vi "MAST_Gage_Acquisition_mod.vi"() -> ()   [LabVIEW 2017]
uses:
  <instrlib>/niHWS/nihws.llb/niHWS Open File Permissions ID.ctl
  <instrlib>/niHWS/nihws.llb/niHWS Set Wfm DBL Attribute ID.ctl
  <instrlib>/niHWS/nihws.llb/niHWS Set Wfm DBL Attribute.vi
  <instrlib>/niHWS/nihws.llb/niHWS Write Analog I16.vi
panel:
  out "Status 2":i32
  out "Error String":string
  in  "One run":bool=TRUE
  out "Waveform Graph":cluster{dbl, dbl, "Data in Volts":i16[]}(graph) caption="Page 1  of  1"
  in  "Save HWS to:":path=path "C:/Users/plasma/Desktop/test.hws"
  in  "Length":dbl=261120.0 min=128.0 max=261120.0
  in  "Start Point":dbl min=-10000000000.0 max=26112000000.0 step=16.0
  in  "Trigger":T1={"Slope"=0, "Level"=20, "Source"=0, "External Range"=2000, "External Coupling"=0, "External"=FALSE, "Disable"=FALSE, "External Impedance"=1} {"External Impedance" items=["50 Ohm", "HiZ"]; "External Coupling" items=["DC", "AC"]; "External Range" min=2000 max=10000 step=8000; "Slope" items=["Rising", "Falling"]; "Level" min=-100 max=100; "Source" min=0 max=64 step=1}
  in  "stop":bool
  in  "Page Size":dbl=32640.0 min=4080.0 step=4080.0
  out "Status":string
  in  "Channels":T2(array[cluster])=[{"Coupling"=0, "Differential Input"=FALSE, "Direct-to-ADC"=FALSE, "Range"=2000, "Impedance"=50, "DC Offset"=0, "Filter"=0}] {"Impedance" min=50 max=1000000 step=999950; "Coupling" items=["DC", "AC"]}
  in  "Acquisition":T3={"Sample Rate"=10000000.0, "Mode"=0, "Depth"=261120.0, "Acquisiton time(s)"=1.0000016, "Trigger Timeout(s)"=10.0, "Trigger Holdoff"=0.0, "Trigger Delay"=0.0, "Clock mode"=enum."Internal"} {"Acquisiton time(s)" min=1.6e-05 max=200.0 step=0.001 format="%_5p"; "Trigger Delay" min=0.0 step=1e-06; "Trigger Holdoff" min=0.0 step=128.0; "Depth" min=16.0 step=16.0; "Mode" items=["Single", "Dual", "Quad", "Octal"]; "Sample Rate" format="%.0p"}
  out "System Name":string
  out "Channel Count":u16
  out "Board Count":u16
  out "System Count":i32
  # "Fetching splitting parameters"
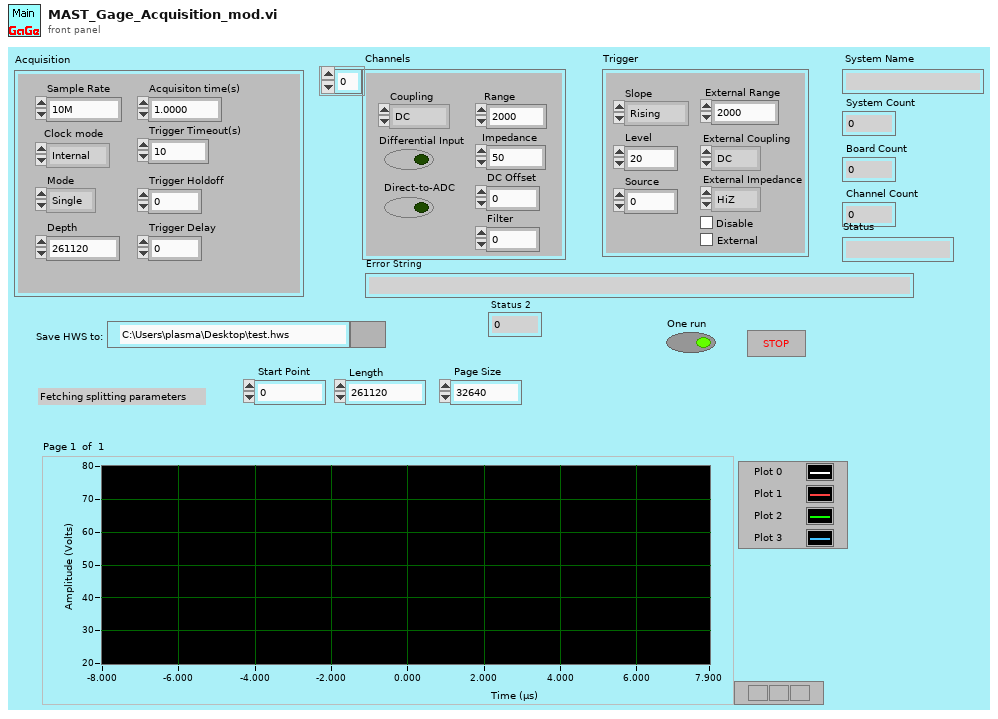
[diagram p1: front panel]
types:
  T1 = cluster{"Slope":u16, "Level":i32, "Source":i32, "External Range":u32, "External Coupling":u16, "External":bool, "Disable":bool, "External Impedance":u16}
  T2 = cluster{"Coupling":u16, "Differential Input":bool, "Direct-to-ADC":bool, "Range":u32, "Impedance":u32, "DC Offset":i32, "Filter":i32}[]
  T3 = cluster{"Sample Rate":dbl, "Mode":u16, "Depth":dbl, "Acquisiton time(s)":dbl, "Trigger Timeout(s)":dbl, "Trigger Holdoff":dbl, "Trigger Delay":dbl, "Clock mode":enum16{"Internal", "External", "Reference"}}
  T4 = typedef "niHWS Open File Permissions ID.ctl" = enum32{"Read Only", "Read/Write Existing", "Read/Write/Create New", "Read/Write/Create New Always"}
  T5 = cluster{"Handle":u32, "Sample size":u32, "Resolution":i32, "Offset":i32, "Channels":u32, "Boards":u32}
  T6 = cluster{"Coupling":u16, "Differential Input":bool, "Direct-to-ADC":bool, "Range":u32, "Impedance":u32, "DC Offset":i32, "Filter":i32}
  T7 = cluster{string, "Differential Input":bool, "Direct-to-ADC":bool, "Range":u32, "Impedance":u32, "DC Offset":i32, "Filter":i32}
  T8 = cluster{"RingText.Text":string, "Level":i32, "Source":i32, "External Range":u32, "RingText.Text":string, "External":bool, "Disable":bool, "RingText.Text":string}
  T9 = cluster{"RingText.Text":string, "Level":i32, "Source":i32, "External Range":u32, "RingText.Text":string, "External":bool, "Disable":bool, "RingText.Text":string}[]
  T10 = cluster{"Sample Rate":dbl, "Clock mode":enum16{"Internal", "External", "Reference"}, "RingText.Text":string, dbl, dbl, dbl, "Trigger Holdoff":dbl, dbl}
  T11 = cluster{"Handle":u32, "Sample Size":u32, "Resolution":i32, "Offset":i32, "Channels":u32, "Boards":u32}
  T12 = typedef "niHWS Set Wfm DBL Attribute ID.ctl" = u32
  T13 = cluster{dbl, dbl, "Data before\n conversion":i16[]}
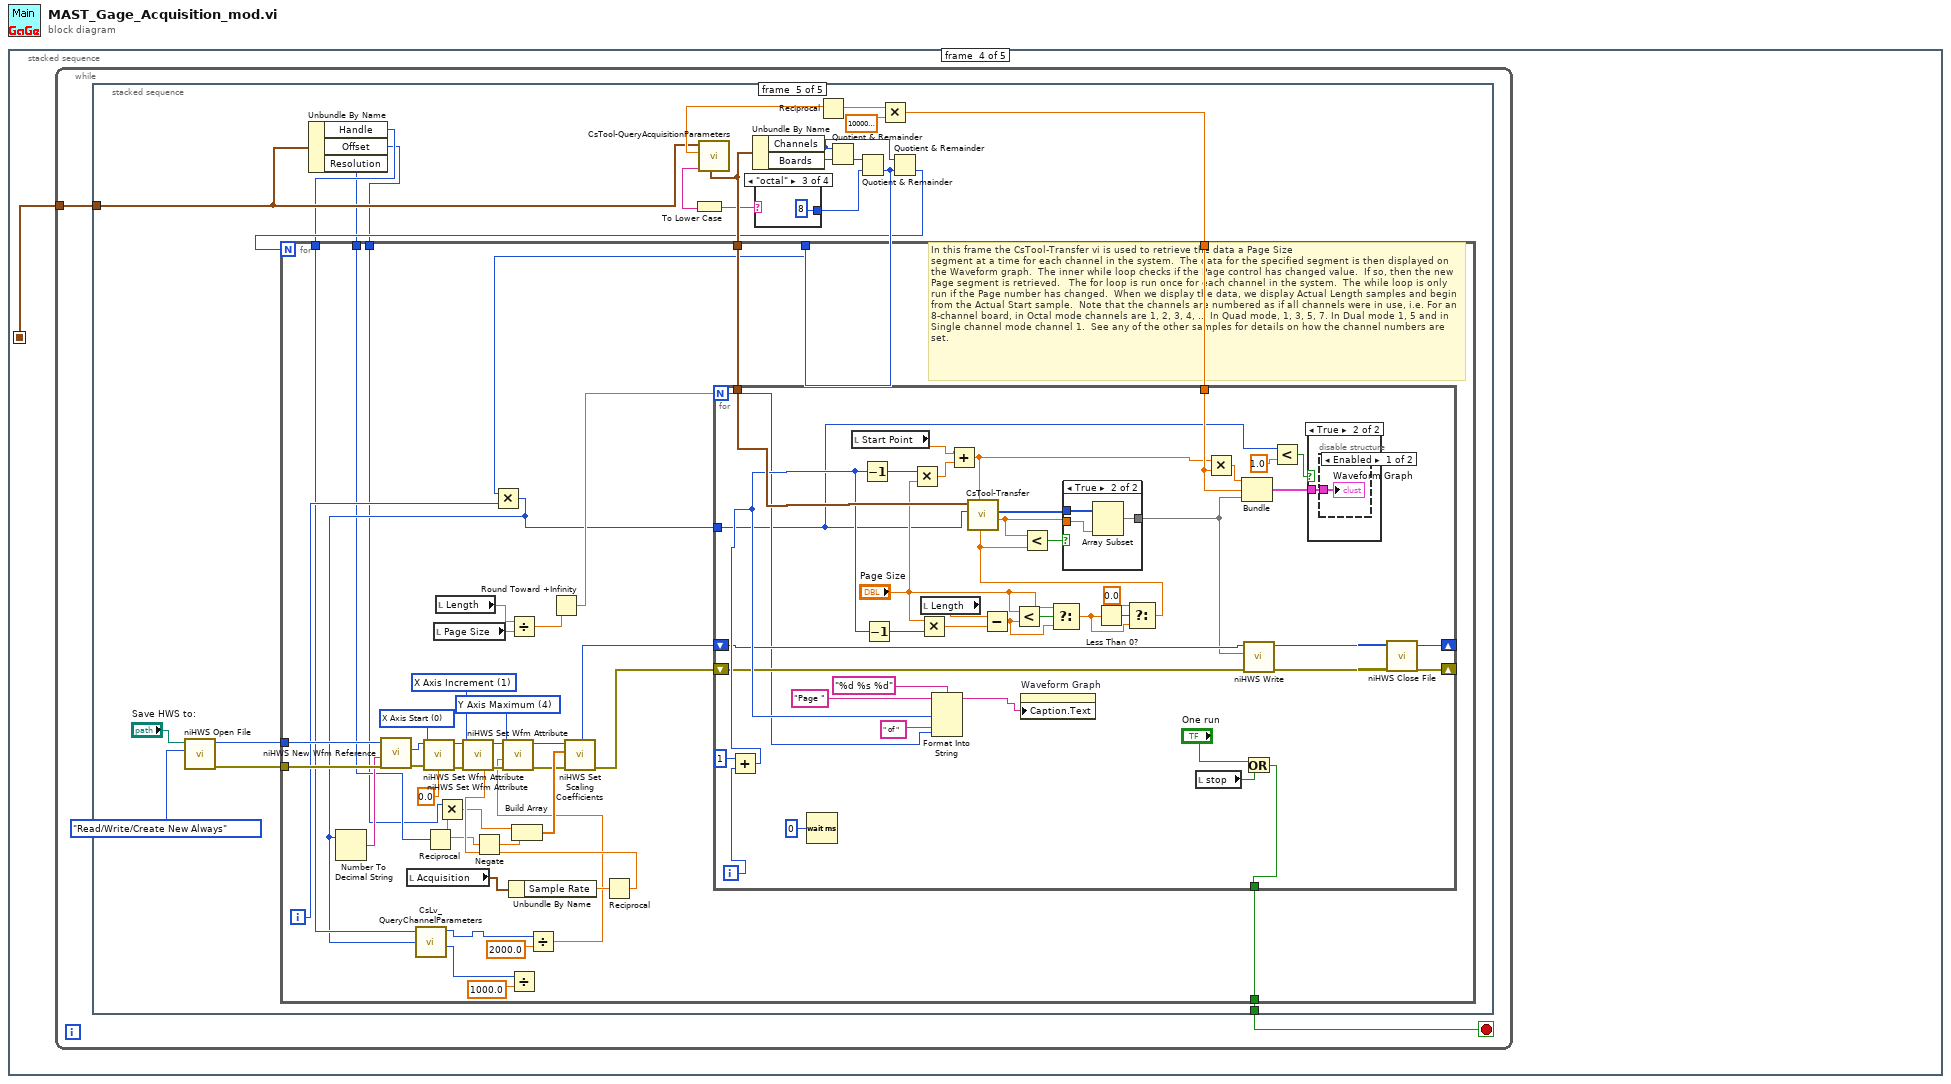
[diagram p0: block diagram]
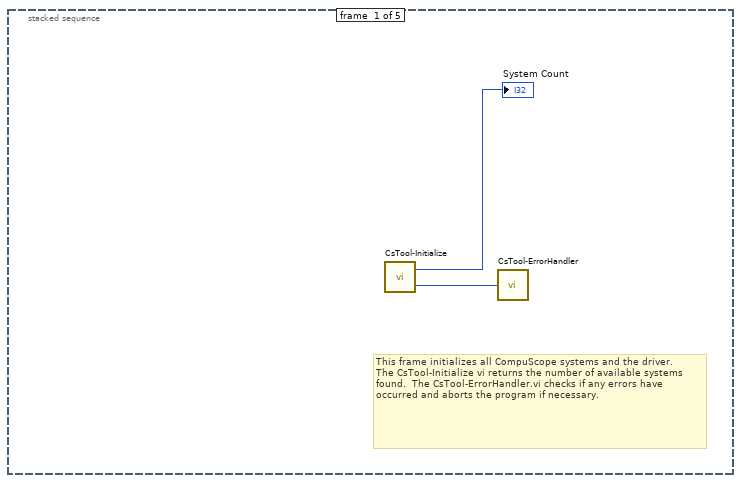
[diagram p2: hidden frame]
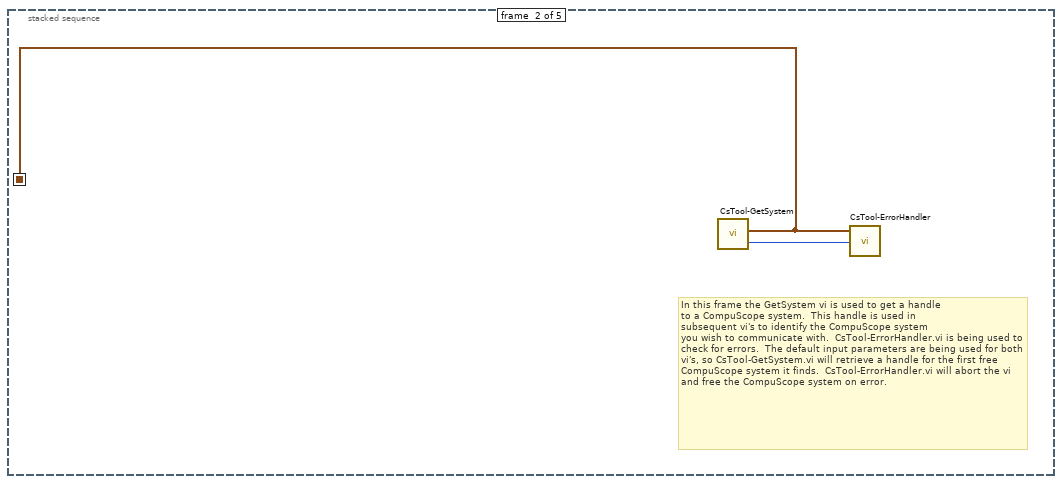
[diagram p3: hidden frame]
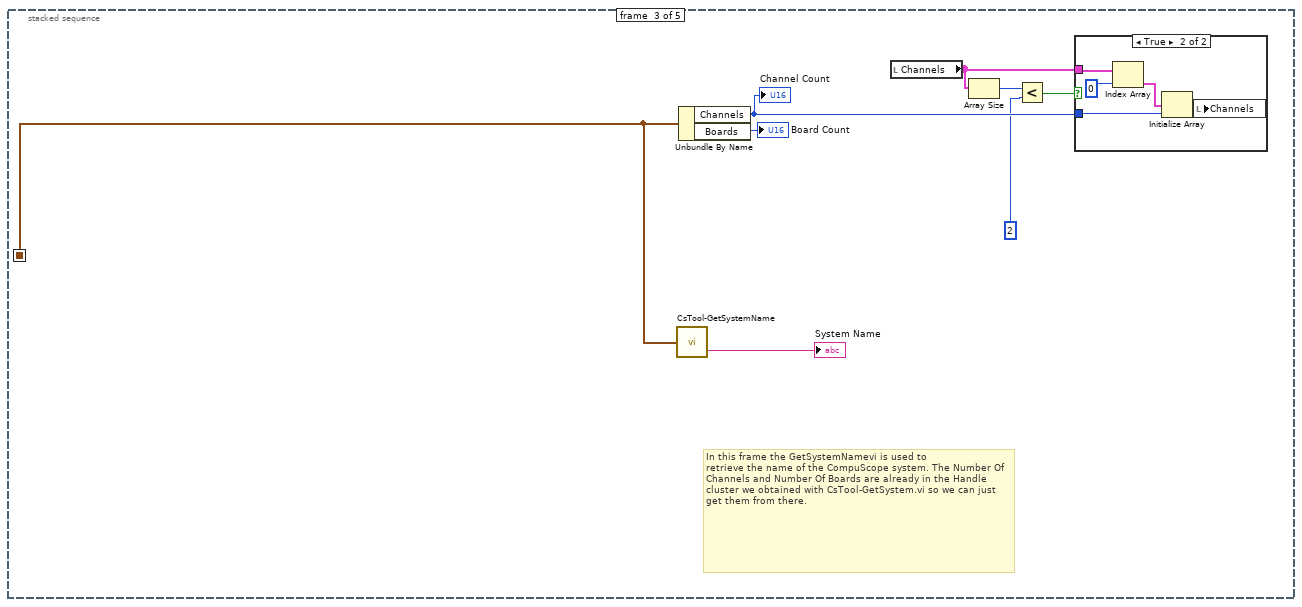
[diagram p4: hidden frame]
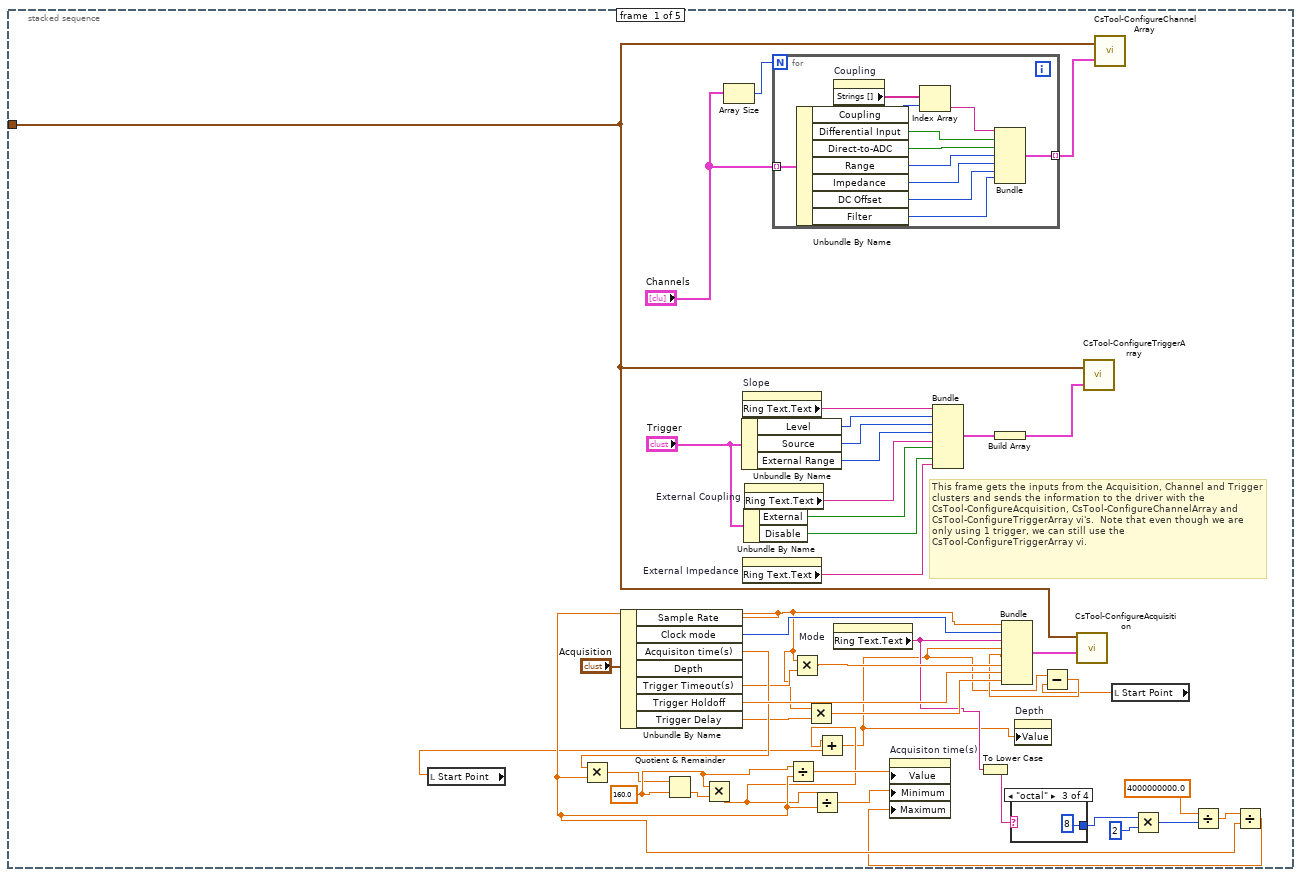
[diagram p6: hidden frame]
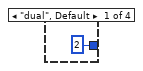
[diagram p7: hidden frame]
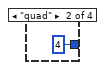
[diagram p8: hidden frame]
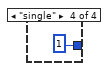
[diagram p9: hidden frame]
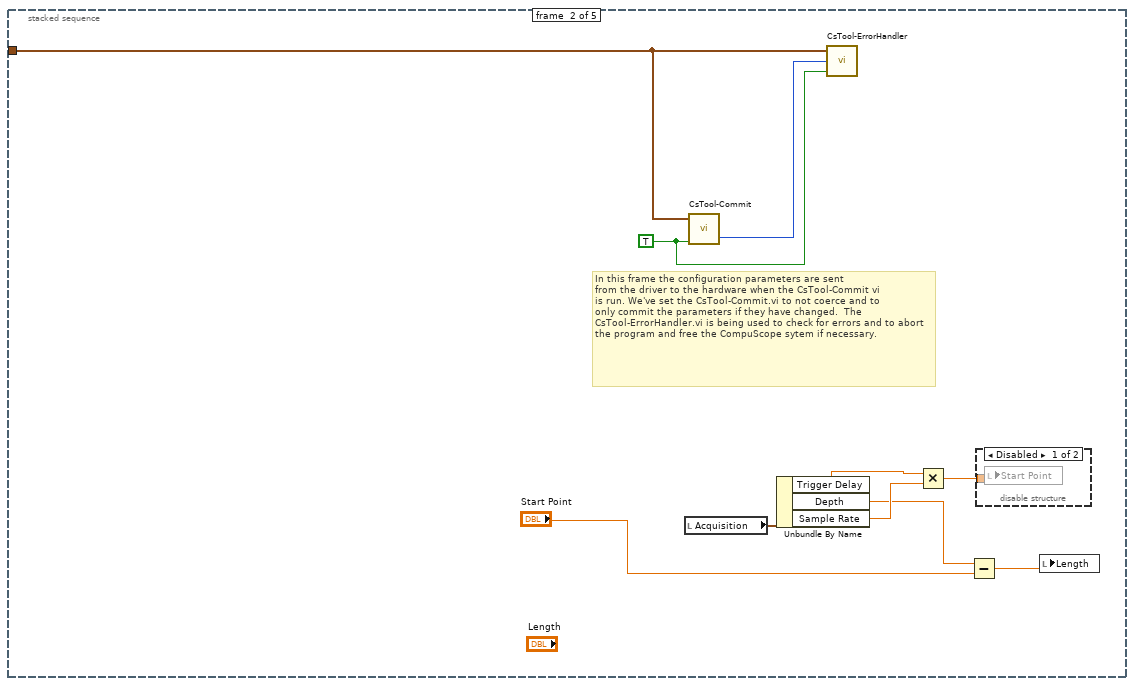
[diagram p10: hidden frame]
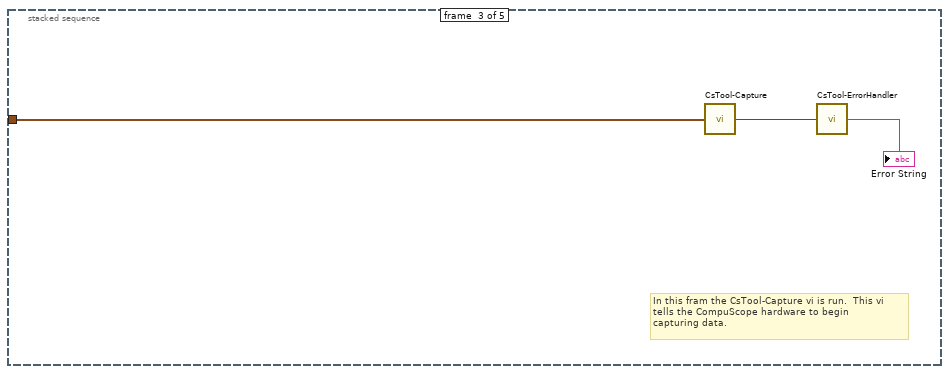
[diagram p12: hidden frame]
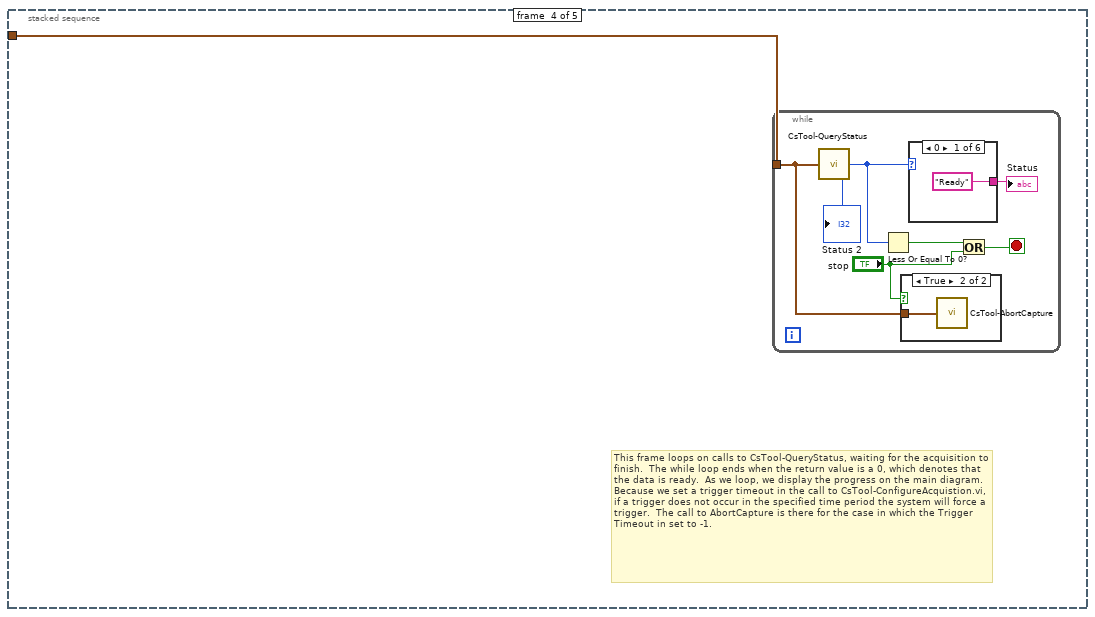
[diagram p13: hidden frame]
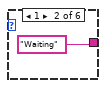
[diagram p15: hidden frame]
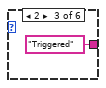
[diagram p16: hidden frame]
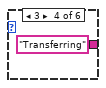
[diagram p17: hidden frame]
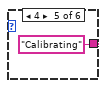
[diagram p18: hidden frame]
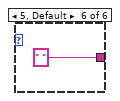
[diagram p19: hidden frame]
diagram:
  n1 = stacked-sequence {
    seq-local: [_ w3 _ _ _] -> [_ _ w11 w18 w225]
    frame #0 {
      # "This frame initializes all CompuScope systems and the driver.\nThe CsTool-Initialize vi returns the number of available systems found.  The CsTool-ErrorHandler.vi checks if any errors have occurred and aborts the program if necessary."
      n2 = call <userlib>:"CsTool-Initialize.vi"() -> ("Error Code"=w2:i32, "Number Of Systems"=→"System Count":i32)
      n3 = call <userlib>:"CsTool-ErrorHandler.vi"("Error Code"=w2) -> ()  [unwired: 2 in, 1 out]
    }
    frame #1 {
      # "In this frame the GetSystem vi is used to get a handle \nto a CompuScope system.  This handle is used in \nsubsequent vi's to identify the CompuScope system \nyou wish to communicate with.  CsTool-ErrorHandler.vi is being used to check for errors.  The default input parameters are being used for both vi's, so CsTool-GetSystem.vi will retrieve a handle for the first free CompuScope system it finds.  CsTool-ErrorHandler.vi will abort the vi and free the CompuScope system on error."
      n4 = call <userlib>:"CsTool-GetSystem.vi"() -> ("Error Code"=w4:i32, "Handle Cluster"=w3:T5)  [unwired: 4 in]
      n5 = call <userlib>:"CsTool-ErrorHandler.vi"("Error Code"=w4, "Handle Cluster"=w3) -> ()  [unwired: 1 in, 1 out]
    }
    frame #2 {
      # "In this frame the GetSystemNamevi is used to\nretrieve the name of the CompuScope system. The Number Of Channels and Number Of Boards are already in the Handle cluster we obtained with CsTool-GetSystem.vi so we can just get them from there."
      n6 = call <userlib>:"CsTool-GetSystemName.vi"("Handle Cluster"=w11) -> ("System Name"=→"System Name":string)  [unwired: 1 out]
      n7 = Unbundle By Name(w11) -> ("Channels"=w10:u32, "Boards"=→"Board Count":u32)
      "Channel Count" <- w10
      n8 = local read "Channels"() -> (w7:T2)
      n9 = Array Size(array=w7) -> (size(s)=w8:i32)
      n10 = Less?(x=w8, y=2) -> (x < y?=w9:bool)
      n11 = case shown="True" w9 {
        tunnel: w7 -> [_ w15]
        tunnel: w10 -> [_ w13]
        frame False {
        }
        frame True {
          n12 = Index Array(array=w15, index=0) -> (element=w14:T6)
          n13 = Initialize Array(w14, w13) -> (w16:T2)
          n14 = local write "Channels"(w16) -> ()
        }
      }
    }
    frame #3 {
      n15 = while {
        tunnel: w18 -> [w20]
        stop <- w19 stop-if-true
        n16 = stacked-sequence {
          tunnel: w20 -> [w59 w86 w91 w93 w110]
          tunnel: [_ _ _ _ w123] -> w19
          frame #0 {
            w43 = 160.0 ("y")
            # "This frame gets the inputs from the Acquisition, Channel and Trigger clusters and sends the information to the driver with the CsTool-ConfigureAcquisition, CsTool-ConfigureChannelArray and CsTool-ConfigureTriggerArray vi's.  Note that even though we are only using 1 trigger, we can still use the CsTool-ConfigureTriggerArray vi."
            n17 = local read "Start Point"() -> (w24:dbl)
            n18 = Unbundle By Name("Acquisition") -> ("Sample Rate"=w29:dbl, "Clock mode"=w45:enum16{"Internal", "External", "Reference"}, "Acquisiton time(s)"=w42:dbl, "Trigger Timeout(s)"=w38:dbl, "Trigger Holdoff"=w48:dbl, "Trigger Delay"=w36:dbl)  [unwired: 1 out]
            n19 = Multiply(x=w42, y=w29) -> (x*y=w41:dbl)
            n20 = Quotient & Remainder(x=w41, y=w43) -> (floor(x/y)=w44:dbl)  [unwired: 1 out]
            n21 = Multiply(x=w43, y=w44) -> (x*y=w25:dbl)
            n22 = Array Size(array="Channels") -> (size(s)=w62:i32)
            n23 = Unbundle By Name("Trigger") -> ("Level"=w57:i32, "Source"=w55:i32, "External Range"=w54:u32)
            n24 = property on="Slope" class="Ring (strict)"() -> ("Ring Text.Text"=w51:string)  [unwired: 2 in, 2 out]
            n25 = property on="External Impedance" class="Ring (strict)"() -> ("Ring Text.Text"=w49:string)  [unwired: 2 in, 2 out]
            n26 = Unbundle By Name("Trigger") -> ("External"=w56:bool, "Disable"=w53:bool)
            n27 = property on="External Coupling" class="Ring (strict)"() -> ("Ring Text.Text"=w50:string)  [unwired: 2 in, 2 out]
            n28 = for {
              N: w62 -> [_]
              tunnel: "Channels" -> [w74] mode=indexing
              tunnel: [w75] -> w60 mode=indexing
              n29 = Unbundle By Name(w74) -> ("Coupling"=w78:u16, "Differential Input"=w73:bool, "Direct-to-ADC"=w72:bool, "Range"=w71:u32, "Impedance"=w70:u32, "DC Offset"=w69:i32, "Filter"=w68:i32)
              n30 = property on="Coupling" class="Ring (strict)"() -> ("Strings []"=w77:string[])  [unwired: 2 in, 2 out]
              n31 = Index Array(array=w77, index=w78) -> (element=w76:string)
              n32 = Bundle(w76, "Differential Input"=w73, "Direct-to-ADC"=w72, "Range"=w71, "Impedance"=w70, "DC Offset"=w69, "Filter"=w68) -> (w75:T7)  [unwired: 1 in]
            }
            n33 = Divide(x=w43, y=w29) -> (x/y=w40:dbl)
            n34 = Multiply(x=w29, y=w38) -> (x*y=w37:dbl)
            n35 = Multiply(x=w29, y=w36) -> (x*y=w35:dbl)
            n36 = Divide(x=w25, y=w29) -> (x/y=w39:dbl)
            n37 = Add(x=w25, y=w24) -> (x+y=w22:dbl)
            n38 = property on="Mode" class="Ring (strict)"() -> ("Ring Text.Text"=w27:string)  [unwired: 2 in, 2 out]
            n39 = Bundle("RingText.Text"=w51, "Level"=w57, "Source"=w55, "External Range"=w54, "RingText.Text"=w50, "External"=w56, "Disable"=w53, "RingText.Text"=w49) -> (w47:T8)  [unwired: 1 in]
            n40 = To Lower Case(string=w27) -> (all lower case string=w26:string)
            n41 = Build Array(w47) -> (w46:T9)
            n42 = case shown="\"octal\"" w26 {
              tunnel: [2 4 8 1] -> w34
              frame "dual", Default {
              }
              frame "quad" {
              }
              frame "octal" {
              }
              frame "single" {
              }
            }
            n43 = property on="Depth" class="DigNum (strict)"("Value"=w22) -> ()  [unwired: 2 in, 2 out]
            n44 = call <userlib>:"CsTool-ConfigureTriggerArray.vi"("Triggers"=w46, "Handle Cluster"=w59) -> ()  [unwired: 1 out]
            n45 = call <userlib>:"CsTool-ConfigureChannelArray.vi"("Channels"=w60, "Handle Cluster"=w59) -> ()  [unwired: 1 out]
            n46 = local read "Start Point"() -> (w21:dbl)
            n47 = Subtract(x=w22, y=w21) -> (x-y=w23:dbl)
            n48 = Bundle("Sample Rate"=w29, "Clock mode"=w45, "RingText.Text"=w27, w22, w23, w37, "Trigger Holdoff"=w48, w35) -> (w63:T10)  [unwired: 1 in]
            n49 = call <userlib>:"CsTool-ConfigureAcquisition.vi"("Handle Cluster"=w59, "Acquisition"=w63) -> ()  [unwired: 3 in, 1 out]
            n50 = Multiply(x=w34, y=2) -> (x*y=w31:i32)
            n51 = Divide(x=4000000000.0, y=w31) -> (x/y=w30:dbl)
            n52 = Divide(x=w30, y=w29) -> (x/y=w28:dbl)
            n53 = property on="Acquisiton time(s)" class="DigNum (strict)"("Value"=w39, "Minimum"=w40, "Maximum"=w28) -> ()  [unwired: 2 in, 2 out]
          }
          frame #1 {
            w87 = TRUE
            # "In this frame the configuration parameters are sent\nfrom the driver to the hardware when the CsTool-Commit vi \nis run. We've set the CsTool-Commit.vi to not coerce and to\nonly commit the parameters if they have changed.  The CsTool-ErrorHandler.vi is being used to check for errors and to abort the program and free the CompuScope sytem if necessary."
            n54 = local read "Acquisition"() -> (w85:T3)
            n55 = call <userlib>:"CsTool-Commit.vi"("OnlyOnChange (t)"=w87, "Handle Cluster"=w86) -> ("Error Code"=w88:i32)  [unwired: 1 in, 1 out]
            n56 = Unbundle By Name(w85) -> ("Trigger Delay"=w84:dbl, "Depth"=w81:dbl, "Sample Rate"=w83:dbl)
            n57 = call <userlib>:"CsTool-ErrorHandler.vi"("StopOnError (true)"=w87, "Error Code"=w88, "Handle Cluster"=w86) -> ()  [unwired: 1 out]
            n58 = Multiply(x=w84, y=w83) -> (x*y=w82:dbl)
            n59 = Subtract(x=w81, y="Start Point") -> (x-y=w80:dbl)
            n60 = disable-structure shown="Disabled" {
              disable-tunnel: w82 -> [w89 _]
              frame Disabled {
                n61 = local write "Start Point"(w89) -> ()
              }
              frame Enabled {
              }
            }
            n62 = local write "Length"(w80) -> ()
          }
          frame #2 {
            # "In this fram the CsTool-Capture vi is run.  This vi\ntells the CompuScope hardware to begin\ncapturing data."
            n63 = call <userlib>:"CsTool-Capture.vi"("Handle Cluster"=w91) -> ("Error Code"=w92:i32)
            n64 = call <userlib>:"CsTool-ErrorHandler.vi"("Error Code"=w92) -> ("Error String"=→"Error String":string)  [unwired: 2 in]
          }
          frame #3 {
            # "This frame loops on calls to CsTool-QueryStatus, waiting for the acquisition to finish.  The while loop ends when the return value is a 0, which denotes that the data is ready.  As we loop, we display the progress on the main diagram.  Because we set a trigger timeout in the call to CsTool-ConfigureAcquistion.vi, if a trigger does not occur in the specified time period the system will force a trigger.  The call to AbortCapture is there for the case in which the Trigger Timeout in set to -1."
            n65 = while {
              tunnel: w93 -> [w95]
              stop <- w96 stop-if-true
              n66 = call <userlib>:"CsTool-QueryStatus.vi"("Handle Cluster"=w95) -> ("Status"=w99:i32)
              "Status 2" <- w99
              n67 = Less Or Equal To 0?(x=w99) -> (x <= 0?=w97:bool)
              n68 = case shown="True" "stop" {
                tunnel: w95 -> [_ w100]
                frame False {
                }
                frame True {
                  n69 = call <userlib>:"CsTool-AbortCapture.vi"("Handle Cluster"=w100) -> ()  [unwired: 1 out]
                }
              }
              n70 = case shown="0" w99 {
                tunnel: ["Ready" "Waiting" "Triggered" "Transferring" "Calibrating" " "] -> w98
                frame 0 {
                }
                frame 1 {
                }
                frame 2 {
                }
                frame 3 {
                }
                frame 4 {
                }
                frame 5, Default {
                }
              }
              "Status" <- w98
              n71 = Or(x=w97, y="stop") -> (x .or. y?=w96:bool)
            }
          }
          frame #4 {
            n72 = call <instrlib>:"niHWS Open File.vi"("permissions (0:read only)"=niHWS_Open_File_Permissions_ID."Read/Write/Create New Always", "file path"="Save HWS to:") -> ("error out"=w113:errorcluster, "file handle"=w114:u32)  [unwired: 8 in]
            n73 = Unbundle By Name(w110) -> ("Handle"=w109:u32, "Offset"=w108:i32, "Resolution"=w107:i32)
            n74 = call <userlib>:"CsTool-QueryAcquisitionParameters.vi"("Handle Cluster"=w110) -> ("Output Handle Cluster"=w128:T11, "Mode"=w117:string, "Sample Rate"=w121:dbl)  [unwired: 8 out]
            n75 = To Lower Case(string=w117) -> (all lower case string=w127:string)
            n76 = Unbundle By Name(w128) -> ("Channels"=w125:u32, "Boards"=w122:u32)
            n77 = case shown="\"octal\"" w127 {
              tunnel: [2 4 8 1] -> w116
              frame "dual", Default {
              }
              frame "quad" {
              }
              frame "octal" {
              }
              frame "single" {
              }
            }
            n78 = Reciprocal(x=w121) -> (1/x=w120:dbl)
            n79 = Quotient & Remainder(x=w125, y=w122) -> (floor(x/y)=w126:u32)  [unwired: 1 out]
            n80 = Quotient & Remainder(x=w126, y=w116) -> (floor(x/y)=w124:u32)  [unwired: 1 out]
            n81 = Multiply(x=w120, y=1000000.0) -> (x*y=w118:dbl)
            n82 = Quotient & Remainder(x=w125, y=w124) -> (floor(x/y)=w111:u32)  [unwired: 1 out]
            n83 = for {
              N: w111 -> [_]
              tunnel: w128 -> [w172]
              tunnel: w124 -> [w171]
              tunnel: [w170] -> w123
              tunnel: w118 -> [w169]
              tunnel: w114 -> [w164]
              tunnel: w113 -> [w163]
              tunnel: w109 -> [w142]
              tunnel: w108 -> [w132]
              tunnel: w107 -> [w133]
              i -> [w151]
              w143 = T12 4 items=["X Axis Start"=0, "X Axis Increment"=1, "Y Axis Minimum"=3, "Y Axis Maximum"=4] ("attribute ID")
              w156 = T12 1 items=["X Axis Start"=0, "X Axis Increment"=1, "Y Axis Minimum"=3, "Y Axis Maximum"=4] ("attribute ID")
              w161 = T12 0 items=["X Axis Start"=0, "X Axis Increment"=1, "Y Axis Minimum"=3, "Y Axis Maximum"=4] ("attribute ID")
              # "In this frame the CsTool-Transfer vi is used to retrieve the data a Page Size \nsegment at a time for each channel in the system.  The data for the specified segment is then displayed on the Waveform graph.  The inner while loop checks if the Page control has changed value.  If so, then the new Page segment is retrieved.   The for loop is run once for each channel in the system.  The while loop is only run if the Page number has changed.  When we display the data, we display Actual Length samples and begin from the Actual Start sample.  Note that the channels are numbered as if all channels were in use, i.e. For an 8-channel board, in Octal mode channels are 1, 2, 3, 4, ... In Quad mode, 1, 3, 5, 7. In Dual mode 1, 5 and in Single channel mode channel 1.  See any of the other samples for details on how the channel numbers are set."
              n84 = local read "Acquisition"() -> (w150:T3)
              n85 = Reciprocal(x=w133) -> (1/x=w130:dbl)
              n86 = local read "Page Size"() -> (w166:dbl)
              n87 = local read "Length"() -> (w168:dbl)
              n88 = Multiply(x=w132, y=w130) -> (x*y=w131:dbl)
              n89 = Negate(x=w130) -> (-x=w129:dbl)
              n90 = Multiply(x=w171, y=w151) -> (x*y=w141:u32)
              n91 = Number To Decimal String(number=w141) -> (decimal integer string=w152:string)  [unwired: 1 in]
              n92 = call <instrlib>:"niHWS New Wfm Reference.vi"("error in (no error)"=w163, "waveform name (empty)"=w152, "file handle in"=w164) -> ("error out"=w159:errorcluster, "waveform reference"=w162:u32)  [unwired: 6 in, 1 out]
              n93 = call <userlib>:"CsLv_QueryChannelParameters.vi"("Channel"=w141, "Handle"=w142) -> ("DC Offset (mV)"=w136:i32, "Input Range (mV)"=w139:u32)  [unwired: 5 out]
              n94 = call-poly <instrlib>:"niHWS Set Wfm Attribute.vi"("error in (no error)"=w159, "attribute value"=0.0, "attribute ID"=w161, "waveform reference in"=w162) -> ("error out"=w158:errorcluster, "waveform reference out"=w157:u32)  [unwired: 6 in]
              n95 = Divide(x=w168, y=w166) -> (x/y=w167:dbl)
              n96 = Unbundle By Name(w150) -> ("Sample Rate"=w149:dbl)
              n97 = Divide(x=w136, y=1000.0) -> ()  [unwired: 1 out]
              n98 = Build Array(w131, w129) -> (w155:dbl[])
              n99 = Divide(x=w139, y=2000.0) -> (x/y=w138:dbl)
              n100 = Round Toward +Infinity(x=w167) -> (ceil(x): smallest int >= x=w165:dbl)
              n101 = Reciprocal(x=w149) -> (1/x=w148:dbl)
              n102 = call-poly <instrlib>:"niHWS Set Wfm Attribute.vi"("error in (no error)"=w158, "attribute value"=w148, "attribute ID"=w156, "waveform reference in"=w157) -> ("error out"=w147:errorcluster, "waveform reference out"=w145:u32)  [unwired: 6 in]
              n103 = call-poly <instrlib>:"niHWS Set Wfm Attribute.vi"("error in (no error)"=w147, "attribute value"=w138, "attribute ID"=w143, "waveform reference in"=w145) -> ("error out"=w146:errorcluster, "waveform reference out"=w144:u32)  [unwired: 6 in]
              n104 = call <instrlib>:"niHWS Set Scaling Coefficients.vi"("error in (no error)"=w146, "coefficient array"=w155, "waveform reference in"=w144) -> ("error out"=w153:errorcluster, "waveform reference out"=w154:u32)  [unwired: 7 in]
              n105 = for {
                N: w165 -> [w176]
                tunnel: w172 -> [w207]
                tunnel: w169 -> [w209]
                tunnel: [w186] -> w170
                shift-right: [w180] -> w135
                shift-left: w154 -> [w182]
                shift-right: [w179] -> w134
                shift-left: w153 -> [w181]
                tunnel: w141 -> [w173]
                i -> [w185]
                n106 = Add(x=1, y=w185) -> (x+y=w184:i32)
                n107 = Wait (ms)(milliseconds to wait=u32 0) -> ()  [unwired: 1 out]
                n108 = local read "Start Point"() -> (w187:dbl)
                n109 = Decrement(x=w184) -> (x-1=w200:i32)
                n110 = Decrement(x=w184) -> (x-1=w191:i32)
                n111 = Multiply(x=w200, y="Page Size") -> (x*y=w199:dbl)
                n112 = Multiply(x="Page Size", y=w191) -> (x*y=w197:dbl)
                n113 = local read "Length"() -> (w198:dbl)
                n114 = Format Into String(format string="%d %s %d", initial string="Page ", w184, " of ", w176) -> (resulting string=w177:string)  [unwired: 1 in, 1 out]
                n115 = Add(x=w187, y=w199) -> (x+y=w203:dbl)
                n116 = Subtract(x=w198, y=w197) -> (x-y=w195:dbl)
                n117 = Less?(x="Page Size", y=w195) -> (x < y?=w196:bool)
                n118 = property on="Waveform Graph" class="WFGraph (strict)"("Caption.Text"=w177) -> ()  [unwired: 2 in, 2 out]
                n119 = Select(t="Page Size", s=w196, f=w195) -> (s? t:f=w192:dbl)
                n120 = Less Than 0?(x=w192) -> (x < 0?=w194:bool)
                n121 = Select(t=0.0, s=w194, f=w192) -> (s? t:f=w189:dbl)
                n122 = call <userlib>:"CsTool-Transfer.vi"("Length (4096)"=w189, "Start (0)"=w203, "Channel (0)"=w173, "Handle Cluster"=w207) -> ("Actual Length"=w188:dbl, "Data before\n conversion"=w201:i16[])  [unwired: 2 in, 2 out]
                n123 = Less?(x=w188, y=w189) -> (x < y?=w202:bool)
                n124 = case shown="True" w202 {
                  tunnel: w201 -> [w216 w219]
                  tunnel: [w216 w218] -> w178
                  tunnel: w188 -> [_ w217]
                  frame False {
                  }
                  frame True {
                    n125 = Array Subset(array=w219, length=w217) -> (w218:i16[])  [unwired: 1 in]
                  }
                }
                n126 = local read "stop"() -> (w208:bool)
                n127 = Multiply(x=w203, y=w209) -> (x*y=w205:dbl)
                n128 = Bundle(w205, w209, "Data before\n conversion"=w178) -> (w204:T13)  [unwired: 1 in]
                n129 = call-poly <instrlib>:"niHWS Write.vi"("error in (no error)"=w181, "data"=w178, "waveform reference in"=w182) -> ("error out"=w179:errorcluster, "waveform reference out"=w180:u32)  [unwired: 7 in]
                n130 = Or(x="One run", y=w208) -> (x .or. y?=w186:bool)
                n131 = Less?(x=w173, y=1.0) -> (x < y?=w175:bool)
                n132 = case shown="True" w175 {
                  tunnel: w204 -> [_ w214]
                  frame False {
                  }
                  frame True {
                    n133 = disable-structure shown="Enabled" {
                      disable-tunnel: w214 -> [w215 _]
                      frame Enabled {
                        "Waveform Graph" <- w215
                      }
                      frame Disabled {
                      }
                    }
                  }
                }
              }
              n134 = call <instrlib>:"niHWS Close File.vi"("error in (no error)"=w134, "file handle"=w135) -> ()  [unwired: 9 in, 1 out]
            }
          }
        }
      }
    }
    frame #4 {
      # "We set the Stop button (actually it's local variable) to False here so when the vi stops the Stop button will not stay depressed."
      # "In this frame, which is reached when the Stop\nis pressed, the CompuScope system is freed by\nrunning the CsTool-FreeSystem vi.  This frees \nany resources used by the system and makes \nit available for another program to use."
      n135 = call <userlib>:"CsTool-FreeSystem.vi"("Handle Cluster"=w225) -> ()  [unwired: 1 out]
      n136 = local write "stop"(FALSE) -> ()
    }
  }
